vi "Write Data.vi"(8 "error in (no error)":errorcluster, 10 "Data":string, 11 "VISA Stream in":refnum<class "Serial Stream.lvclass">) -> (0 "error out":errorcluster, 3 "VISA Stream out":refnum<class "Serial Stream.lvclass">)   [LabVIEW 2020, in "Stream-Serial.lvlib" / "Serial Stream.lvclass"]
uses:
  Serial Stream.lvclass
  C:/Program Files (x86)/National Instruments/LabVIEW 2020/vi.lib/IlluminatedG/lv-stream/stream/Stream.lvclass
  Serial Stream.lvclass/Serial Stream.ctl
  <vilib>/IlluminatedG/lv-stream/stream/Stream.lvclass
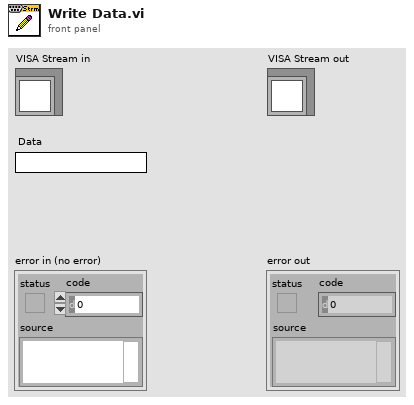
[diagram p1: front panel]
types:
  T1 = typedef "Stream.lvlib/Mode.ctl" = enum16{"Raw", "Buffered", "LineTerm"}
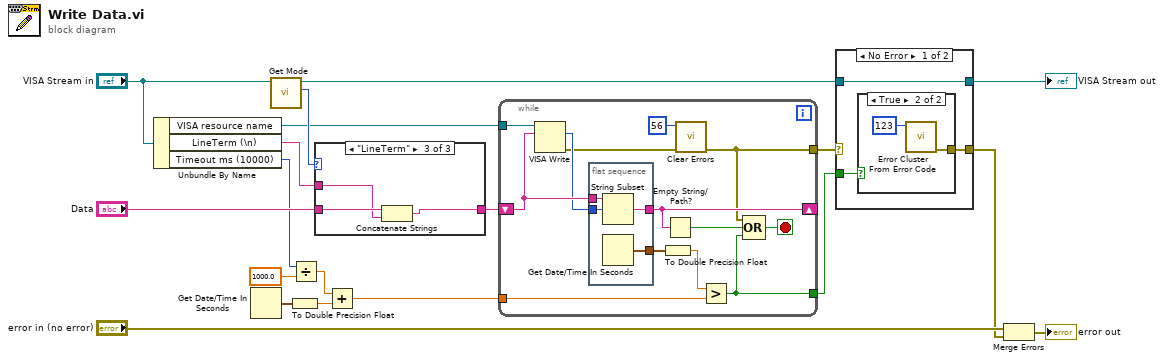
[diagram p0: block diagram]
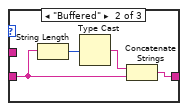
[diagram p3: hidden frame]
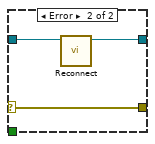
[diagram p5: hidden frame]
diagram:
  n1 = Unbundle By Name("VISA Stream in") -> ("VISA resource name"=w5:refnum<visa-resource-name>, "LineTerm (\\n)"=w16:string, "Timeout ms (10000)"=w13:i32)
  n2 = Get Date/Time In Seconds() -> (seconds since 1Jan1904=w14:timestamp)
  n3 = call <vilib>:"Get Mode.vi"("Stream in"="VISA Stream in") -> ("Mode"=w17:T1, "Stream out"=w9:refnum<class "Serial Stream.lvclass">)  [unwired: 8 in, 1 out]
  n4 = To Double Precision Float(number=w14) -> (double precision float=w11:dbl)
  n5 = Divide(x=w13, y=1000.0) -> (x/y=w10:dbl)
  n6 = case shown="\"LineTerm\"" w17 {
    tunnel: w16 -> [_ _ w26]
    tunnel: "Data" -> [w20 w22 w27]
    tunnel: [w20 w21 w25] -> w1
    frame "Raw" {
    }
    frame "Buffered" {
      n7 = String Length(string=w22) -> (length=w24:i32)
      n8 = Type Cast(x=w24) -> (*(type *) &x=w23:string)  [unwired: 1 in]
      n9 = Concatenate Strings(w23, w22) -> (w21:string)
    }
    frame "LineTerm" {
      n10 = Concatenate Strings(w27, w26) -> (w25:string)
    }
  }
  n11 = Add(x=w10, y=w11) -> (x+y=w4:dbl)
  n12 = while {
    tunnel: w5 -> [w40]
    tunnel: w4 -> [w36]
    shift-right: [w32] -> _
    shift-left: w1 -> [w39]
    tunnel: [w34] -> w3
    tunnel: [w29] -> w2
    stop <- w33 stop-if-true
    n13 = VISA Write(VISA resource name=w40, write buffer=w39) -> (return count=w38:u32, error out=w30:errorcluster)  [unwired: 1 in, 1 out]
    n14 = flat-sequence {
      tunnel: w39 -> [w44]
      tunnel: [w43] -> w32
      tunnel: w38 -> [w42]
      tunnel: [w41] -> w37
      frame #0 {
        n15 = String Subset(string=w44, offset (0)=w42) -> (substring=w43:string)  [unwired: 1 in]
        n16 = Get Date/Time In Seconds() -> (seconds since 1Jan1904=w41:timestamp)
      }
    }
    n17 = To Double Precision Float(number=w37) -> (double precision float=w35:dbl)
    n18 = Empty String/Path?(string/path=w32) -> (empty?=w31:bool)
    n19 = call <vilib>:"Clear Errors.vi"("error in (no error)"=w30, "specific error code to clear (0: all)"=56) -> ("error out"=w29:errorcluster)  [unwired: 4 in, 1 out]
    n20 = Greater?(x=w35, y=w36) -> (0:w34:bool)
    n21 = Compound Arithmetic op=OR(w29, w31, w34) -> (w33:bool)
  }
  n22 = case shown="No Error" w2 {
    selector: w2 -> [_ w50]
    tunnel: w3 -> [w47 _]
    tunnel: w9 -> [w46 w52]
    tunnel: [w46 w51] -> w8
    tunnel: [w45 w50] -> w6
    frame No Error {
      n23 = case shown="True" w47 {
        tunnel: [_ w48] -> w45
        frame False {
        }
        frame True {
          n24 = call <vilib>:"Error Cluster From Error Code.vi"("error code (0)"=123) -> ("error out"=w48:errorcluster)  [unwired: 8 in]
        }
      }
    }
    frame Error {
      n25 = call "Reconnect.vi"("Serial Stream in"=w52) -> ("Serial Stream out"=w51:refnum<class "Serial Stream.lvclass">)  [unwired: 9 in, 1 out]
    }
  }
  "VISA Stream out" <- w8
  n26 = Merge Errors("error in (no error)", w6) -> (→"error out":errorcluster)
